vi "Export to PDF.vi"(8 "error in":errorcluster, 10 "Path Out":path, 11 "LG_WordReportGeneration.lvlib:Word_Report":refnum<class "Word_Report.lvclass">) -> (0 "error out":errorcluster, 3 "LG_WordReportGeneration.lvlib:Word_Report":refnum<class "Word_Report.lvclass">)   [LabVIEW 2018, in "WordReportGeneration.lvlib" / "Word_Report.lvclass"]
uses:
  Word_Report.lvclass
  C:/Program Files (x86)/National Instruments/LabVIEW 2018/vi.lib/Utility/NIReport.llb/NI_report.lvclass
  <vilib>/Utility/NIReport.llb/Word/NI_Word.lvclass
  <vilib>/Utility/NIReport.llb/Excel/NI_Excel.lvclass
  <vilib>/Utility/NIReport.llb/NI_report.lvclass
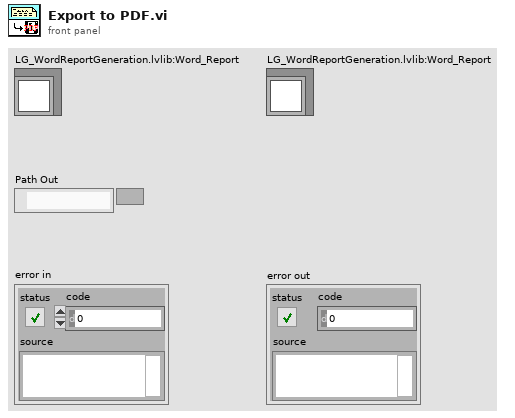
[diagram p1: front panel]
types:
  T1 = typedef "NI_ReportGenerationCore.lvlib/Report Type.ctl" = enum16{"HTML", "Word", "Excel"}
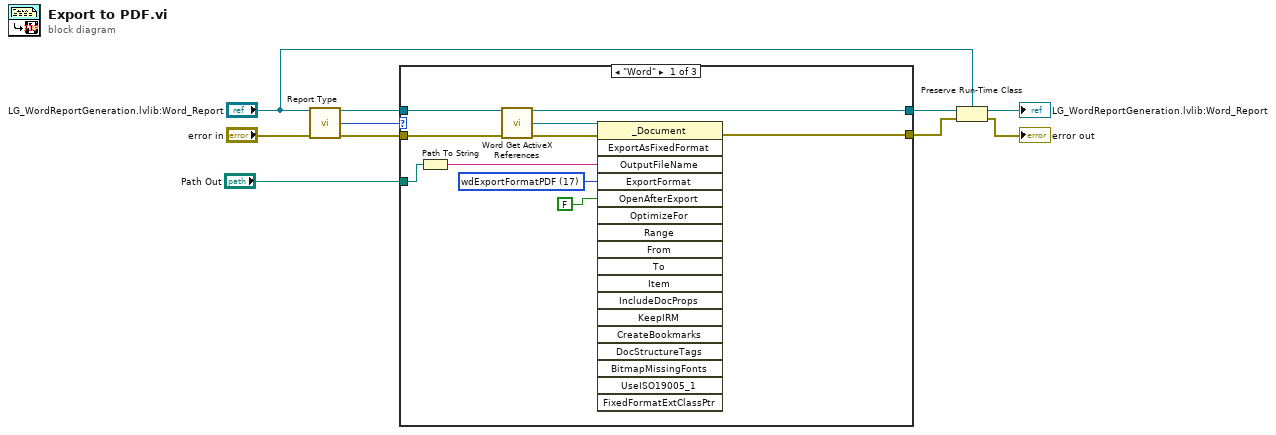
[diagram p0: block diagram]
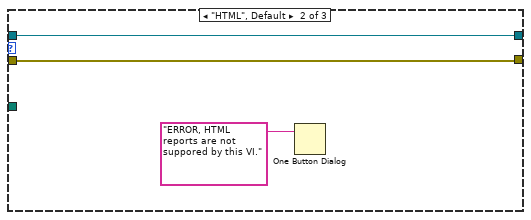
[diagram p2: hidden frame]
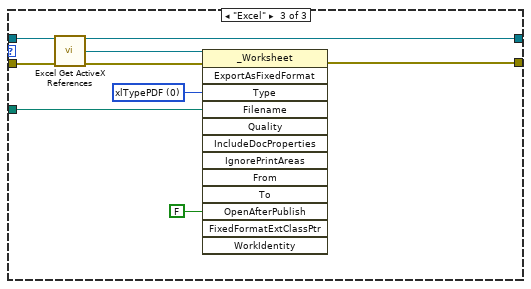
[diagram p3: hidden frame]
diagram:
  n1 = call-dynamic "Report Type.vi"("report in"="LG_WordReportGeneration.lvlib:Word_Report", "error in (no error)"="error in") -> ("report out"=w10:refnum<class "Word_Report.lvclass">, "report type"=w6:T1, "error out"=w8:errorcluster)  [unwired: 11 in]
  n2 = case shown="\"Word\"" w6 {
    tunnel: w10 -> [w20 w23 w31]
    tunnel: "Path Out" -> [w17 _ w30]
    tunnel: [w19 w23 w28] -> w9
    tunnel: w8 -> [w14 w21 w27]
    tunnel: [w12 w21 w25] -> w2
    frame "Word" {
      w15 = 17 items=["wdExportFormatPDF"=17, "wdExportFormatXPS"=18] ("ExportFormat")
      n3 = Path To String(path=w17) -> (string=w16:string)
      n4 = call <vilib>:"Word Get ActiveX References.vi"("report in"=w20, "error in (no error)"=w14) -> ("report out"=w19:refnum<class "NI_report.lvclass">, "Word._Document"=w18:refnum<k7>, "error out"=w13:errorcluster)  [unwired: 7 in, 4 out]
      n5 = invoke class="_Document" method="ExportAsFixedFormat"(reference=w18, error in=w13, "OutputFileName"=w16, "ExportFormat"=w15, "OpenAfterExport"=FALSE) -> (error out=w12:errorcluster)  [unwired: 13 in, 17 out]
    }
    frame "HTML", Default {
      n6 = One Button Dialog(message="ERROR, HTML reports are not suppored by this VI.") -> ()  [unwired: 1 in, 1 out]
    }
    frame "Excel" {
      w24 = 0 items=["xlTypePDF", "xlTypeXPS"] ("Type")
      n7 = call <vilib>:"Excel Get ActiveX References.vi"("report in"=w31, "error in (no error)"=w27) -> ("report out"=w28:refnum<class "NI_report.lvclass">, "Excel._Worksheet"=w32:refnum<k7>, "error out"=w26:errorcluster)  [unwired: 7 in, 4 out]
      n8 = invoke class="_Worksheet" method="ExportAsFixedFormat"(reference=w32, error in=w26, "Type"=w24, "Filename"=w30, "OpenAfterPublish"=FALSE) -> (error out=w25:errorcluster)  [unwired: 8 in, 12 out]
    }
  }
  n9 = Preserve Run-Time Class(object in=w9, error in=w2, 2:"LG_WordReportGeneration.lvlib:Word_Report") -> (object out=→"LG_WordReportGeneration.lvlib:Word_Report":refnum<class "Word_Report.lvclass">, error out=→"error out":errorcluster)
